vi "FeedbackDecode_PickROI.vi"(3 "RespStrRef":refnum<vi>) -> ()   [LabVIEW 2020]
uses:
  <vilib>/Utility/miscctls.llb/LVPoint32TypeDef.ctl
  FeedbackDecode_Globals.vi
  <vilib>/imath/engines/lvmath2/RunTimeEngine/IndexRead/NIMS M($,S).vi
  <instcachedir>/0/NIMS M($,S)_3E5749BBB62E49528D4765A77F1F6D98.lvgen/NIMS M($,S)_3E5749BBB62E49528D4765A77F1F6D98_000.vi
  <vilib>/imath/engines/lvmath2/RunTimeEngine/IndexRead/NIMS V(S).vi
  <instcachedir>/0/NIMS V(S)_0488751826AF41519A22953C041130DC.lvgen/NIMS V(S)_0488751826AF41519A22953C041130DC_000.vi
  <vilib>/imath/engines/lvmath2/RunTimeEngine/BuiltInFunctions/abs/NIMS_abs(signed).vi
  <instcachedir>/0/NIMS_abs(signed)_C4FCB8E6058B49B797C7C8D53CA5F6EC.lvgen/NIMS_abs(signed)_C4FCB8E6058B49B797C7C8D53CA5F6EC_001.vi
  <vilib>/imath/engines/lvmath2/RunTimeEngine/IndexReplace/NIMS M($,S)=V.vi
  <instcachedir>/0/NIMS M($,S)=V_85A28EB895514E96A13A10261726EE3A.lvgen/NIMS M($,S)=V_85A28EB895514E96A13A10261726EE3A_001.vi
  <vilib>/imath/engines/lvmath2/RunTimeEngine/ErrorHandling/NIMS_Create Error From Enums.vi
  <vilib>/imath/engines/lvmath2/RunTimeEngine/BuiltInFunctions/sum/NIMS_sum(GM,Sca).vi
  <instcachedir>/0/NIMS_sum(GM,Sca)_BFF867FCA20B40888962313BF0DBA2C0.lvgen/NIMS_sum(GM,Sca)_BFF867FCA20B40888962313BF0DBA2C0_001.vi
  <vilib>/imath/engines/lvmath2/RunTimeEngine/BuiltInFunctions/min/1 input/NIMS_min(RV).vi
  <instcachedir>/0/NIMS_min(RV)_EE2DD3E2888846108C5160A664B67832.lvgen/NIMS_min(RV)_EE2DD3E2888846108C5160A664B67832_000.vi
  <vilib>/imath/engines/lvmath2/RunTimeEngine/NodeEndStatement/NIMS_NodeEndStatement_Output.vi
  <instcachedir>/0/NIMS_NodeEndStatement_Output_53EC0D466D134D7ABD903AC30B43404B.lvgen/NIMS_NodeEndStatement_Output_53EC0D466D134D7ABD903AC30B43404B_010.vi
  <vilib>/imath/engines/lvmath2/RunTimeEngine/ErrorHandling/NIMS_Finalize Error.vi
panel:
  out "Coords":T1
  out "Output Color":u32(colorbox)
  out "PickROIStr":string
  in  "Abort":bool
  out "Click":bool=TRUE
  out "CursClck":dbl[](array[numeric])
  out "SensorRow":dbl
  out "StrSensor":string
  out "StrSensation":string
  in  "NoPercept":bool
  in  "Other":bool
  out "RGBtbl":dbl[][](array[numeric])
  in  "Array 2":dbl[][](array[numeric])
  out "SensStr":string[][](array[string])
  in  "Array":string[][](array[string])
  out "Sensor Cluster":T2
  in  "Pressure":bool
  in  "Motion":bool
  out "ErMsg":bool
  out "Count":i32
  out "Resample":bool
  out "RGB":dbl[](array[numeric])
  out "Red":u8
  out "Green":u8
  out "Blue":u8
  out "2D Picture":picture
  in  "Submit":bool
  # "Click on color region where the sensation occurs :"
  # "Describe the sensation (choose one):"
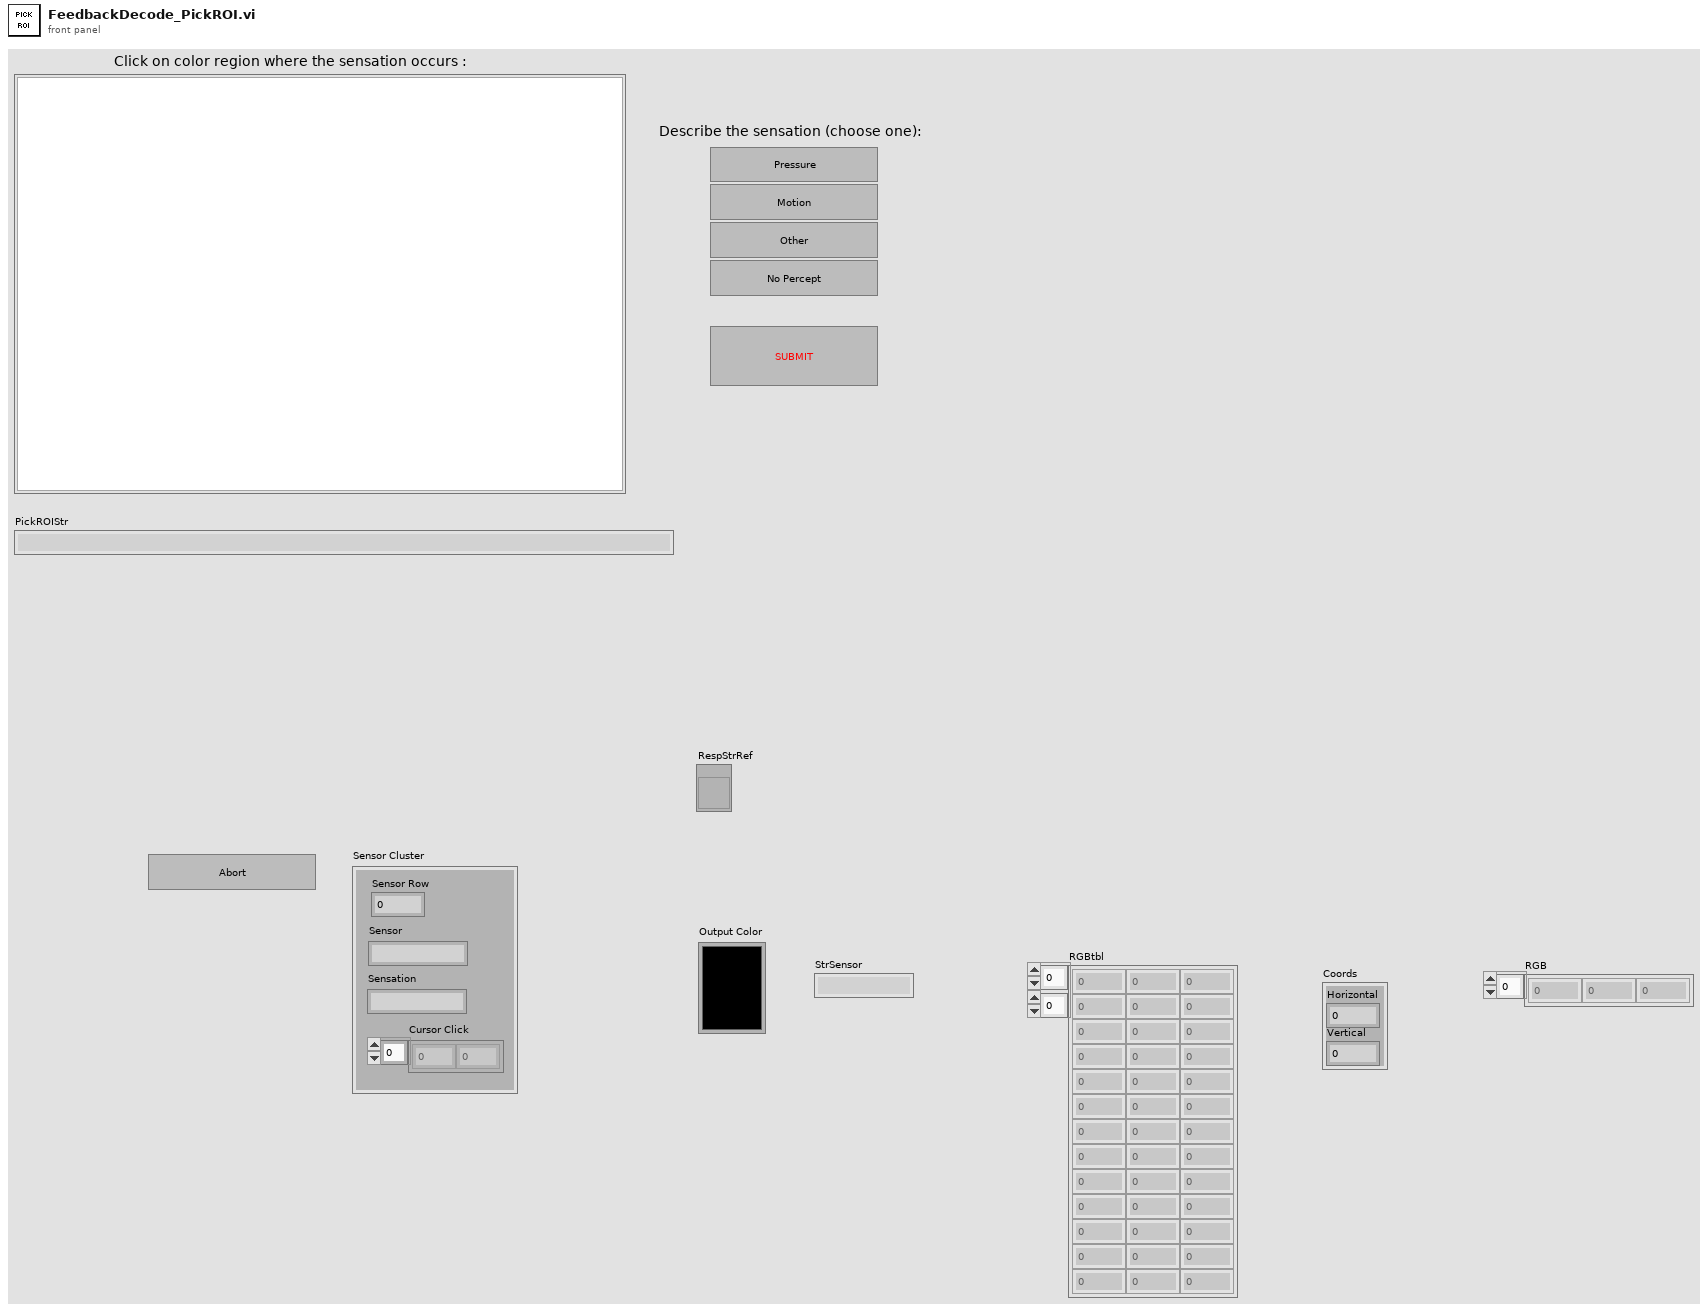
[diagram p1: front panel]
types:
  T1 = typedef "LVPoint32TypeDef.ctl" = cluster{"Horizontal":i32, "Vertical":i32}
  T2 = cluster{"Sensor Row":dbl, "Sensor":string, "Sensation":string, "Cursor Click":dbl[]}
  T3 = typedef "imagedata.ctl" = cluster{"image type":i32, "image depth":i32, "image":u8[], "mask":u8[], "colors":u32[], "Rectangle":cluster{"left":i16, "top":i16, "right":i16, "bottom":i16}}
  T4 = typedef "LVPositionTypeDef.ctl" = cluster{"Left":i32, "Top":i32}
  T5 = cluster{"SensorRow":dbl, "StrSensor":string, "StrSensation":string, "CursClck":dbl[]}
  T6 = enum32{"Invalid", "Standard", "Closed", "Hidden", "Minimized", "Maximized"}
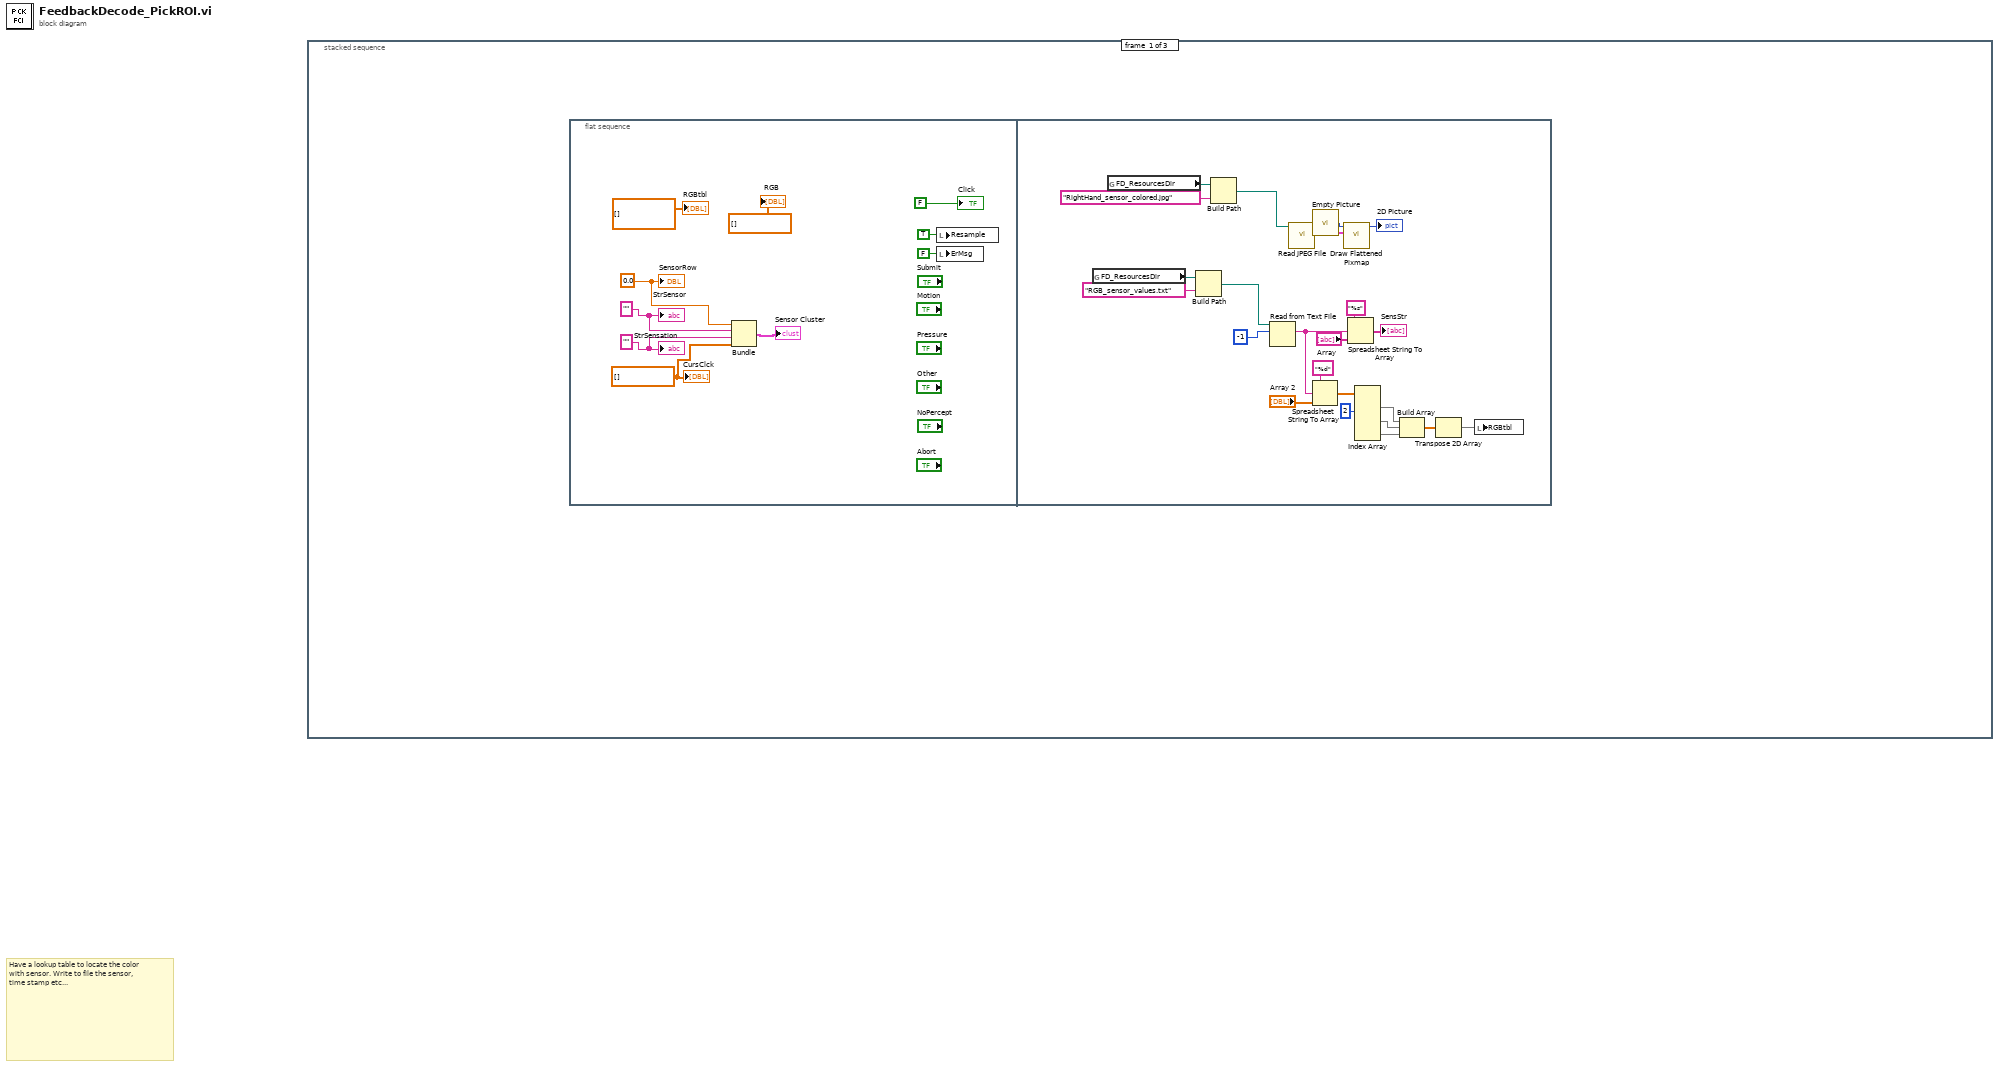
[diagram p0: block diagram]
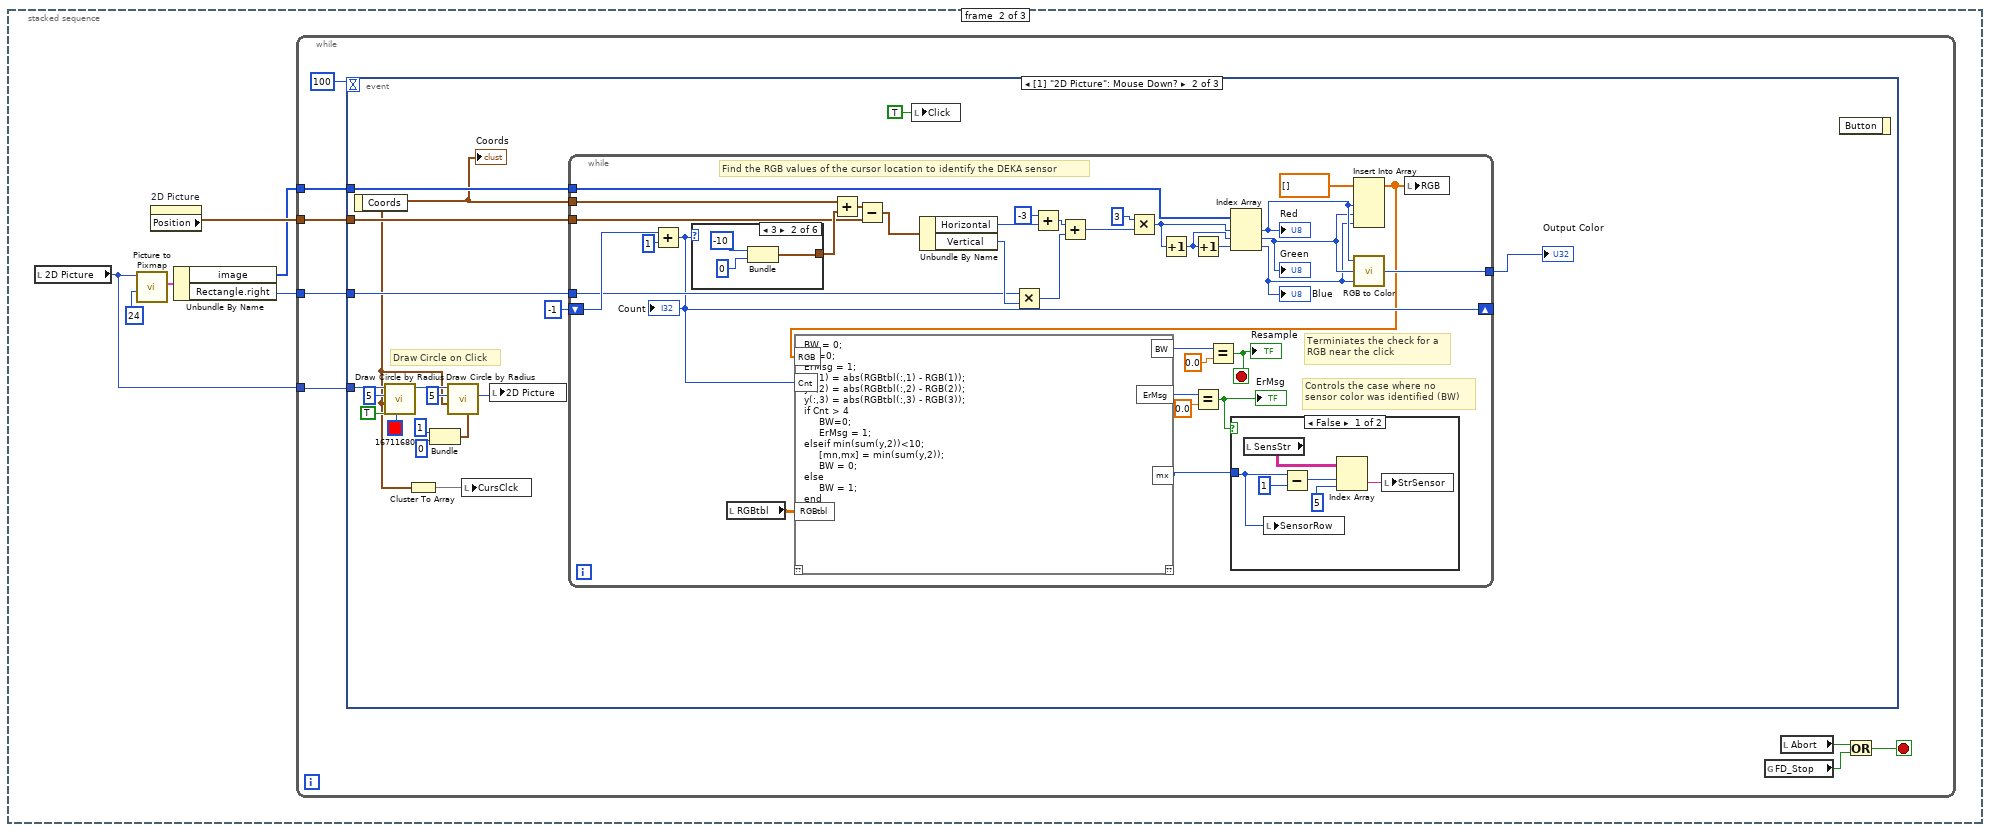
[diagram p2: hidden frame]
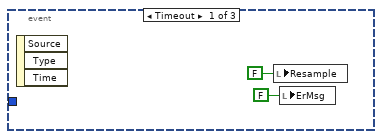
[diagram p3: hidden frame]
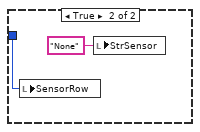
[diagram p4: hidden frame]
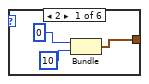
[diagram p5: hidden frame]
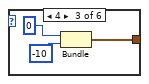
[diagram p6: hidden frame]
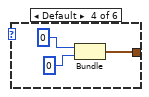
[diagram p7: hidden frame]
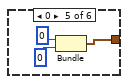
[diagram p8: hidden frame]
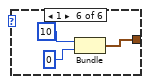
[diagram p9: hidden frame]
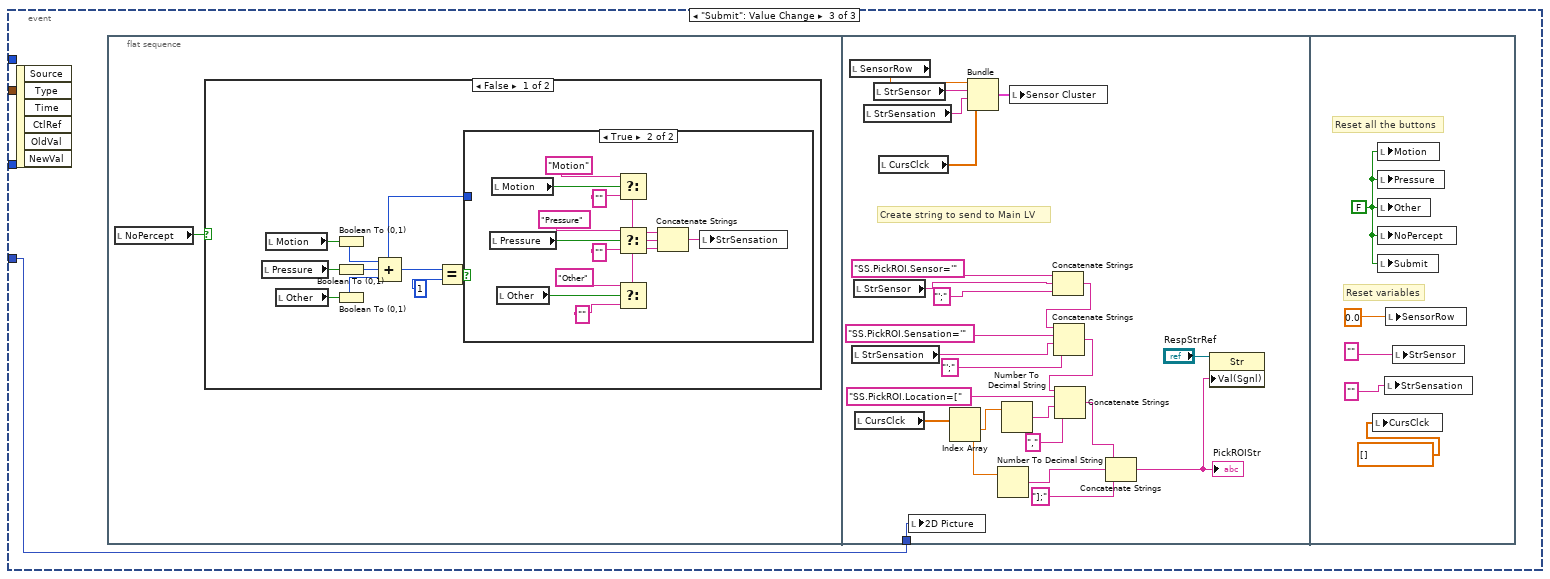
[diagram p10: hidden frame]
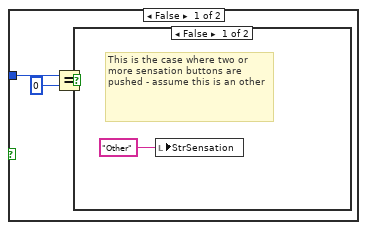
[diagram p11: hidden frame]
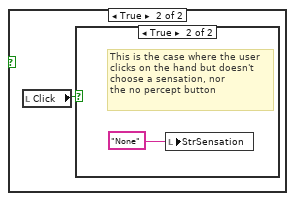
[diagram p12: hidden frame]
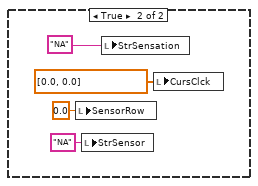
[diagram p14: hidden frame]
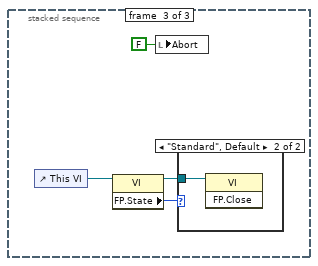
[diagram p15: hidden frame]
diagram:
  # "Have a lookup table to locate the color with sensor. Write to file the sensor, time stamp etc..."
  n1 = stacked-sequence {
    frame #0 {
      n2 = flat-sequence {
        frame #0 {
          w3 = dbl[] [] ("RGB Array")
          w6 = 0.0
          w5 = ""
          w4 = ""
          n3 = Bundle(w6, w5, w4, "RGB Array"=w3) -> (→"Sensor Cluster":cluster{dbl, string, string, "RGB Array":dbl[]})  [unwired: 1 in]
          n4 = local write "Resample"(TRUE ("Resample")) -> ()
          n5 = local write "ErMsg"(FALSE ("ErMsg")) -> ()
          "RGB" <- dbl[] [] ("RGB Array")
          "RGBtbl" <- dbl[][] [] ("RGB Array")
          "StrSensation" <- w4
          "StrSensor" <- w5
          "SensorRow" <- w6
          "CursClck" <- w3
          "Click" <- FALSE ("Resample")
        }
        frame #1 {
          n6 = global read "FeedbackDecode_Globals.vi" "FD_ResourcesDir"() -> (w13:path)
          n7 = global read "FeedbackDecode_Globals.vi" "FD_ResourcesDir"() -> (w15:path)
          n8 = Build Path(base path=w13, name or relative path="RGB_sensor_values.txt") -> (appended path=w11:path)
          n9 = Build Path(base path=w15, name or relative path="RightHand_sensor_colored.jpg") -> (appended path=w14:path)
          n10 = Read from Text File(file (use dialog)=w11, count=-1) -> (text=w22:string)  [unwired: 2 in, 3 out]
          n11 = call <vilib>:"Read JPEG File.vi"("path to JPEG file"=w14) -> ("image data"=w31:T3)  [unwired: 8 in, 2 out]
          n12 = Spreadsheet String To Array(format string="%d", spreadsheet string=w22, array type (2D Dbl)="Array 2") -> (array=w28:dbl[][])  [unwired: 1 in]
          n13 = call "Empty Picture"() -> ("empty picture"=w32:picture)
          n14 = call <vilib>:"Draw Flattened Pixmap.vi"("image data"=w31, "picture"=w32) -> ("new picture"=→"2D Picture":picture)  [unwired: 7 in]
          n15 = Spreadsheet String To Array(format string="%s", spreadsheet string=w22, array type (2D Dbl)="Array") -> (array=→"SensStr":string[][])  [unwired: 1 in]
          n16 = Index Array(array=w28, index (col) #1=2 ("disabled index (col)")) -> (element #1=w30:dbl[], element #2=w25:dbl[], element #3=w24:dbl[])  [unwired: 5 in]
          n17 = Build Array(w30, w25, w24) -> (w26:dbl[][])
          n18 = Transpose 2D Array(2D array=w26) -> (transposed array=w29:dbl[][])
          n19 = local write "RGBtbl"(w29) -> ()
        }
      }
    }
    frame #1 {
      n20 = local read "2D Picture"() -> (w34:picture)
      n21 = call <vilib>:"Picture to Pixmap.vi"("depth"=24, "picture"=w34) -> ("image data"=w38:T3)  [unwired: 8 in, 1 out]
      n22 = property on="2D Picture" class="Pict"() -> ("Position"=w37:T4)  [unwired: 2 in, 2 out]
      n23 = Unbundle By Name(w38) -> ("image"=w35:u8[], "Rectangle.right"=w36:i16)
      n24 = while {
        tunnel: w37 -> [w46]
        tunnel: w36 -> [w45]
        tunnel: w35 -> [w44]
        tunnel: w34 -> [w43]
        stop <- w40 stop-if-true
        n25 = event shown="[1] \"2D Picture\": Mouse Down?" {
          selector: _ -> [_ _ _]
          dyn-events: _ -> [_ _ _]
          timeout: 100 -> [_ _ _]
          tunnel: w46 -> [_ w67 _]
          tunnel: w45 -> [_ w66 _]
          tunnel: w44 -> [_ w65 _]
          tunnel: w43 -> [_ w62 w329]
          event Timeout {
            n26 = event-data() -> ()  [unwired: 1 in, 3 out]
            n27 = local write "Resample"(FALSE) -> ()
            n28 = local write "ErMsg"(FALSE) -> ()
          }
          event "2D Picture": Mouse Down? {
            # "Draw Circle on Click"
            n29 = event-data() -> ("Coords"=w51:T1)  [unwired: 1 in]
            "Coords" <- w51
            n30 = call <vilib>:"Draw Circle by Radius.vi"("color(black)"=u32 16711680, "fill?(F)"=TRUE, "pixel center"=w51, "radius"=i16 5, "picture"=w62) -> ("new picture"=w56:picture)  [unwired: 6 in]
            n31 = Cluster To Array(cluster=w51) -> (array=w52:i32[])
            n32 = Bundle(1, 0) -> (w54:cluster{i32, i32})  [unwired: 1 in]
            n33 = call <vilib>:"Draw Circle by Radius.vi"("pen"=w54, "pixel center"=w51, "radius"=i16 5, "picture"=w56) -> ("new picture"=w55:picture)  [unwired: 7 in]
            n34 = local write "CursClck"(w52) -> ()
            n35 = local write "2D Picture"(w55) -> ()
            n36 = while {
              tunnel: w67 -> [w80]
              tunnel: w51 -> [w74]
              tunnel: w66 -> [w79]
              tunnel: w65 -> [w94]
              tunnel: [w93] -> w64
              shift-right: [w72] -> _
              shift-left: -1 -> [w87]
              stop <- w82 stop-if-true
              # "Controls the case where no\nsensor color was identified (BW)"
              # "Terminiates the check for a\nRGB near the click"
              # "Find the RGB values of the cursor location to identify the DEKA sensor"
              n37 = Add(x=w87, y=1) -> (x+y=w72:i32)
              "Count" <- w72
              n38 = case shown="3" w72 {
                tunnel: [w311 w314 w317 w320 w323 w326] -> w81
                frame 2 {
                  n39 = Bundle(0, 10) -> (w311:cluster{i32, i32})  [unwired: 1 in]
                }
                frame 3 {
                  n40 = Bundle(-10, 0) -> (w314:cluster{i32, i32})  [unwired: 1 in]
                }
                frame 4 {
                  n41 = Bundle(0, -10) -> (w317:cluster{i32, i32})  [unwired: 1 in]
                }
                frame Default {
                  n42 = Bundle(0, 0) -> (w320:cluster{i32, i32})  [unwired: 1 in]
                }
                frame 0 {
                  n43 = Bundle(0, 0) -> (w323:cluster{i32, i32})  [unwired: 1 in]
                }
                frame 1 {
                  n44 = Bundle(10, 0) -> (w326:cluster{i32, i32})  [unwired: 1 in]
                }
              }
              n45 = local read "RGBtbl"() -> (w73:dbl[][])
              n46 = Add(x=w74, y=w81) -> (x+y=w84:T1)
              n47 = Subtract(x=w84, y=w80) -> (x-y=w85:T1)
              n48 = Unbundle By Name(w85) -> ("Horizontal"=w77:i32, "Vertical"=w95:i32)
              n49 = Multiply(x=w79, y=w95) -> (x*y=w101:i32)
              n50 = Add(x=-3, y=w77) -> (x+y=w78:i32)
              n51 = Add(x=w78, y=w101) -> (x+y=w100:i32)
              n52 = Multiply(x=3, y=w100) -> (x*y=w98:i32)
              n53 = Increment(x=w98) -> (x+1=w97:i32)
              n54 = Increment(x=w97) -> (x+1=w96:i32)
              n55 = Index Array(array=w94, index #1=w98, index #2=w97, index #3=w96) -> (element #1=w91:u8, element #2=w90:u8, element #3=w89:u8)
              "Red" <- w91
              "Green" <- w90
              "Blue" <- w89
              n56 = Insert Into Array(array=dbl[] [] ("Horizontal"), new element #1=w91, new element #2=w90, new element #3=w89) -> (w69:dbl[])  [unwired: 1 in]
              n57 = mathscript code="BW = 0;\nmx=0;\nErMsg = 1;\ny(:,1) = abs(RGBtbl(:,1) - RGB(1));\ny(:,2) = abs(RGBtbl(:,2) - RGB(2));\ny(:,3) = abs(RGBtbl(:,3) - RGB(3));\nif Cnt > 4\n     BW=0;\n     ErMsg = 1;\nelseif min(sum(y,2))<10;\n     [mn,mx] = min(sum(y,2));\n     BW = 0;\nelse \n     BW = 1;\nend"("RGBtbl"=w73, "RGB"=w69, "Cnt"=w72) -> ("BW"=w71:i32, "ErMsg"=w70:i32, "mx"=w68:i32)  [unwired: 1 in, 1 out]
              n58 = Equal?(x=w70, y=0.0) -> (x = y?=w75:bool)
              "ErMsg" <- w75
              n59 = Equal?(x=w71, y=0.0) -> (x = y?=w82:bool)
              "Resample" <- w82
              n60 = case shown="False" w75 {
                tunnel: w68 -> [w303 w310]
                frame False {
                  n61 = local read "SensStr"() -> (w307:string[][])
                  n62 = local write "SensorRow"(w303) -> ()
                  n63 = Subtract(x=w303, y=u8 1) -> (x-y=w306:i32)
                  n64 = Index Array(array=w307, index (row)=w306, index (col)=5 ("disabled index (col)")) -> (element=w304:string)
                  n65 = local write "StrSensor"(w304) -> ()
                }
                frame True {
                  n66 = local write "SensorRow"(w310) -> ()
                  n67 = local write "StrSensor"("None" ("StrSensor")) -> ()
                }
              }
              n68 = call <vilib>:"RGB to Color.vi"("B"=w89, "G"=w90, "R"=w91) -> ("Color"=w93:u32)
              n69 = local write "RGB"(w69) -> ()
            }
            "Output Color" <- w64
            n70 = local write "Click"(TRUE ("Click")) -> ()
            n71 = event-data() -> ()  [unwired: 2 in, 1 out]
          }
          event "Submit": Value Change {
            n72 = event-data() -> ()  [unwired: 1 in, 6 out]
            n73 = flat-sequence {
              tunnel: w329 -> [w382]
              frame #0 {
                n74 = local read "NoPercept"() -> (w330:bool)
                n75 = case shown="False" w330 {
                  frame False {
                    n76 = local read "Pressure"() -> (w334:bool)
                    n77 = local read "Motion"() -> (w335:bool)
                    n78 = local read "Other"() -> (w339:bool)
                    n79 = Boolean To (0,1)(Boolean=w335) -> (0, 1=w336:i16)
                    n80 = Boolean To (0,1)(Boolean=w334) -> (0, 1=w337:i16)
                    n81 = Boolean To (0,1)(Boolean=w339) -> (0, 1=w338:i16)
                    n82 = Compound Arithmetic op=ADD(w336, w337, w338) -> (w331:i16)
                    n83 = Equal?(x=w331, y=i16 1) -> (x = y?=w332:bool)
                    n84 = case shown="True" w332 {
                      tunnel: w331 -> [w342 _]
                      frame False {
                        n85 = Equal?(x=w342, y=i16 0) -> (x = y?=w340:bool)
                        n86 = case shown="False" w340 {
                          frame False {
                            # "This is the case where two or more sensation buttons are pushed - assume this is an other"
                            n87 = local write "StrSensation"("Other") -> ()
                          }
                          frame True {
                            n88 = local read "Click"() -> (w344:bool)
                            n89 = case shown="True" w344 {
                              frame False {
                                # "This is the case where\n the user doesn't choose a\nnything or click on the hand"
                              }
                              frame True {
                                # "This is the case where the user \nclicks on the hand but doesn't \nchoose a sensation, nor\nthe no percept button"
                                n90 = local write "StrSensation"("None") -> ()
                              }
                            }
                          }
                        }
                      }
                      frame True {
                        n91 = local read "Pressure"() -> (w354:bool)
                        n92 = local read "Motion"() -> (w346:bool)
                        n93 = local read "Other"() -> (w353:bool)
                        n94 = Select(t="Motion", s=w346, f="") -> (s? t:f=w355:string)
                        n95 = Select(t="Pressure", s=w354, f="") -> (s? t:f=w356:string)
                        n96 = Select(t="Other", s=w353, f="") -> (s? t:f=w357:string)
                        n97 = Concatenate Strings(w355, w356, w357) -> (w358:string)
                        n98 = local write "StrSensation"(w358) -> ()
                      }
                    }
                  }
                  frame True {
                    n99 = local write "SensorRow"(0.0 ("SensorRow")) -> ()
                    n100 = local write "StrSensor"("NA" ("StrSensor")) -> ()
                    n101 = local write "StrSensation"("NA") -> ()
                    n102 = local write "CursClck"(dbl[] [0.0, 0.0] ("CursClck")) -> ()
                  }
                }
              }
              frame #1 {
                # "Create string to send to Main LV"
                n103 = local read "SensorRow"() -> (w384:dbl)
                n104 = local read "StrSensation"() -> (w376:string)
                n105 = local read "StrSensor"() -> (w379:string)
                n106 = local read "CursClck"() -> (w372:dbl[])
                n107 = local read "StrSensation"() -> (w385:string)
                n108 = local read "StrSensor"() -> (w386:string)
                n109 = local read "CursClck"() -> (w383:dbl[])
                n110 = local write "2D Picture"(w382) -> ()
                n111 = Index Array(array=w372) -> (element #1=w371:dbl, element #2=w366:dbl)  [unwired: 2 in]
                n112 = Bundle("SensorRow"=w384, "StrSensor"=w386, "StrSensation"=w385, "CursClck"=w383) -> (w387:T5)  [unwired: 1 in]
                n113 = Number To Decimal String(number=w366) -> (decimal integer string=w367:string)  [unwired: 1 in]
                n114 = Number To Decimal String(number=w371) -> (decimal integer string=w370:string)  [unwired: 1 in]
                n115 = local write "Sensor Cluster"(w387) -> ()
                n116 = Concatenate Strings("SS.PickROI.Sensor='", w379, "';") -> (w378:string)
                n117 = Concatenate Strings(w378, "SS.PickROI.Sensation='", w376, "';") -> (w374:string)
                n118 = Concatenate Strings(w374, "SS.PickROI.Location=[", w370, ",") -> (w365:string)
                n119 = Concatenate Strings(w365, w367, "];") -> (w363:string)
                "PickROIStr" <- w363
                n120 = property on="Property Node" class="Str"(reference="RespStrRef", "Val(Sgnl)"=w363) -> ()  [unwired: 1 in, 2 out]
              }
              frame #2 {
                w392 = FALSE ("Motion")
                # "Reset variables"
                # "Reset all the buttons"
                n121 = local write "CursClck"(dbl[] [] ("RGB Array")) -> ()
                n122 = local write "Motion"(w392) -> ()
                n123 = local write "Pressure"(w392) -> ()
                n124 = local write "Other"(w392) -> ()
                n125 = local write "NoPercept"(w392) -> ()
                n126 = local write "Submit"(w392) -> ()
                n127 = local write "StrSensation"("") -> ()
                n128 = local write "SensorRow"(0.0) -> ()
                n129 = local write "StrSensor"("") -> ()
              }
            }
          }
        }
        n130 = global read "FeedbackDecode_Globals.vi" "FD_Stop"() -> (w41:bool)
        n131 = local read "Abort"() -> (w42:bool)
        n132 = Or(x=w42, y=w41) -> (x .or. y?=w40:bool)
      }
    }
    frame #2 {
      n133 = control-ref of="This VI"() -> (w393:refnum<vi>)
      n134 = property class="VI"(reference=w393) -> (reference out=w394:refnum<vi>, "FP.State"=w395:T6)  [unwired: 1 in, 1 out]
      n135 = local write "Abort"(FALSE ("Abort")) -> ()
      n136 = case shown="\"Standard\", Default" w395 {
        tunnel: w394 -> [_ w397]
        frame "Closed" {
        }
        frame "Standard", Default {
          n137 = invoke class="VI" method="FP.Close"(reference=w397) -> ()  [unwired: 2 in, 3 out]
        }
      }
    }
  }
